vi "AWS-S3-DestroyClient.vi"(0 "Mini AWS S3 API":refnum<class "AWS-S3-MiniAPI.lvclass">, 11 "error in":errorcluster) -> (15 "error out":errorcluster)   [LabVIEW 2012, in "AWS-S3-MiniAPI.lvclass"]
uses:
  AWS-S3-MiniAPI.lvclass
  AWS-S3-MiniAPI.lvclass/AWS-S3-MiniAPI.ctl
  C:/Users/Jack/cla-2013-deployment-automation-and-release-engineering-in-labview/Deployment/AWS-SDK/AWSSDK.dll
  AWS-SDK/AWSSDK.dll
panel:
  # "Inputs"
  # "Outputs"
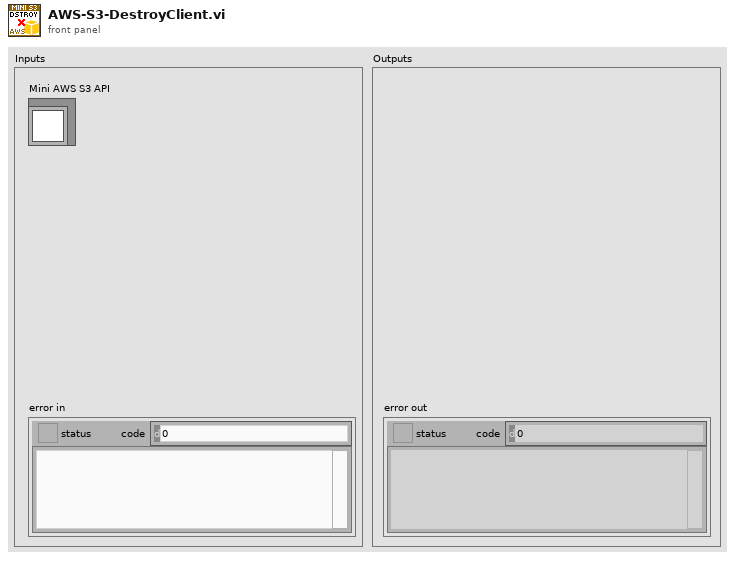
[diagram p1: front panel]
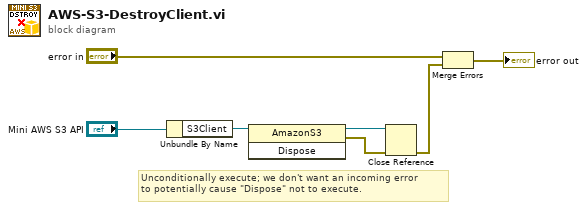
[diagram p0: block diagram]
diagram:
  # "Unconditionally execute; we don't want an incoming error\nto potentially cause \"Dispose\" not to execute."
  n1 = Unbundle By Name("Mini AWS S3 API") -> ("S3Client"=w7:refnum<k24>)
  n2 = invoke class="AmazonS3" method="Dispose"(reference=w7) -> (reference out=w4:refnum<k24>, error out=w3:errorcluster)  [unwired: 2 in, 1 out]
  n3 = Close Reference(reference=w4, error in (no error)=w3) -> (error out=w2:errorcluster)
  n4 = Merge Errors("error in", w2) -> (→"error out":errorcluster)
